vi "MeanShift.vi"(8 "error in":errorcluster) -> (0 "error out":errorcluster, 3 "out":refnum<class "MeanShift.lvclass">)   [LabVIEW 2020]
doc: "Mean shift clustering using a flat kernel.\n\n Mean shift clustering aims to discover \"blobs\" in a smooth density of\n samples. It is a centroid-based algorithm, which works by updating\n candidates for centroids to be the mean of the points within a given\n region. These candidates are then filtered in a post-processing stage to\n eliminate near-duplicates to form the final set of centroids.\n\n Seeding is performed using a binning technique for scalability.\n\n Read more in the :ref:`User Guide <mean_shift>`.\n\n Parameters\n ----------\n bandwidth : float, default=None\n Bandwidth used in the RBF kernel.\n\n If not given, the bandwidth is estimated using\n sklearn.cluster.estimate_bandwidth; see the documentation for that\n function for hints on scalability (see also the Notes, below).\n\n seeds : array-like of shape (n_samples, n_features), default=None\n Seeds used to initialize kernels. If not set,\n the seeds are calculated by clustering.get_bin_seeds\n with bandwidth as the grid size and default values for\n other parameters.\n\n bin_seeding : bool, default=False\n If true, initial kernel locations are not locations of all\n points, but rather the location of the discretized version of\n points, where points are binned onto a grid whose coarseness\n corresponds to the bandwidth. Setting this option to True will speed\n up the algorithm because fewer seeds will be initialized.\n The default value is False.\n Ignored if seeds argument is not None.\n\n min_bin_freq : int, default=1\n To speed up the algorithm, accept only those bins with at least\n min_bin_freq points as seeds.\n\n cluster_all : bool, default=True\n If true, then all points are clustered, even those orphans that are\n not within any kernel. Orphans are assigned to the nearest kernel.\n If false, then orphans are given cluster label -1.\n\n n_jobs : int, default=None\n The number of jobs to use for the computation. This works by computing\n each of the n_init runs in parallel.\n\n ``None`` means 1 unless in a :obj:`joblib.parallel_backend` context.\n ``-1`` means using all processors. See :term:`Glossary <n_jobs>`\n for more details.\n\n max_iter : int, default=300\n Maximum number of iterations, per seed point before the clustering\n operation terminates (for that seed point), if has not converged yet.\n\n .. versionadded:: 0.22\n\n Attributes\n ----------\n cluster_centers_ : ndarray of shape (n_clusters, n_features)\n Coordinates of cluster centers.\n\n labels_ : ndarray of shape (n_samples,)\n Labels of each point.\n\n n_iter_ : int\n Maximum number of iterations performed on each seed.\n\n .. versionadded:: 0.22\n\n \nAvailable methods:\nGet Attributes\nGet Params\nSet Params"
uses:
  MeanShift.lvclass
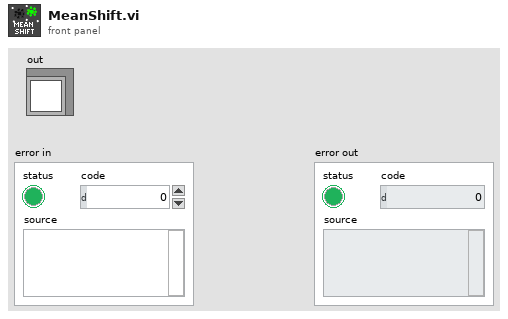
[diagram p1: front panel]
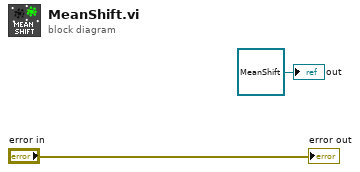
[diagram p0: block diagram]
diagram:
  "out" <- refnum<class "MeanShift.lvclass"> refnum ("model")
  "error out" <- "error in"
